vi "Generate Raw Data.vi"(8 "Error In":errorcluster, 10 "Matrix":u32[][](array[colorbox]), 11 "Display In":refnum<class "Neopixel - Host.lvclass">) -> (0 "Error Out":errorcluster, 2 "Raw Data":u8[](array[numeric]), 3 "Display Out":refnum<class "Neopixel - Host.lvclass">)   [LabVIEW 2021, in "Neopixel - Host.lvclass"]
uses:
  Neopixel - Host.lvclass
  Neopixel - Host.lvclass/Neopixel - Host.ctl
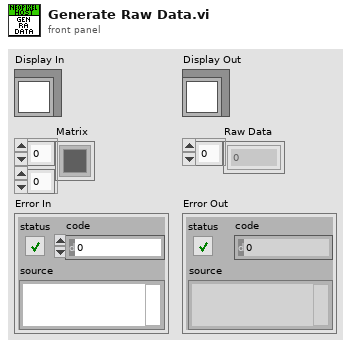
[diagram p1: front panel]
types:
  T1 = typedef "Neopixel - Host.lvclass/RGB Gains.ctl" = cluster{"Red":sgl, "Green":sgl, "Blue":sgl}
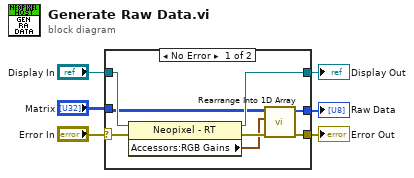
[diagram p0: block diagram]
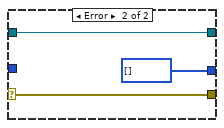
[diagram p2: hidden frame]
diagram:
  n1 = case shown="No Error" "Error In" {
    selector: "Error In" -> [w13 w16]
    tunnel: "Matrix" -> [w8 _]
    tunnel: [w10 w16] -> w4
    tunnel: [w9 u8[] []] -> w3
    tunnel: "Display In" -> [w14 w15]
    tunnel: [w12 w15] -> w1
    frame No Error {
      n2 = property class="Neopixel - RT"(reference=w14, error in=w13) -> (reference out=w12:refnum<class "Neopixel - Host.lvclass">, error out=w11:errorcluster, "Accessors:RGB Gains"=w7:T1)
      n3 = call "Rearrange Into 1D Array.vi"("Error In"=w11, "RGB Gains"=w7, "Matrix"=w8) -> ("Error Out"=w10:errorcluster, "Raw Data"=w9:u8[])  [unwired: 7 in]
    }
    frame Error {
    }
  }
  "Raw Data" <- w3
  "Error Out" <- w4
  "Display Out" <- w1
